vi "create test channels.vi"() -> (0 "error out":errorcluster, 1 "names":string[](array[string]), 2 "Array":refnum<class "EIP Tags Channel.lvclass">[](array[class]), 3 "EthernetIP configuration out":refnum<class "EIP Tags Configuration.lvclass">)   [LabVIEW 2013, in "EthernetIP tests.lvlib"]
uses:
  EthernetIP tests.lvlib
  channel/EIP Tags Channel.lvclass
  configuration/EIP Tags Configuration.lvclass
  configuration/eip tag types.ctl
  <vilib>/NI/Configuration Framework/serializable configuration/NISE_CEF_serializable configuration.lvclass
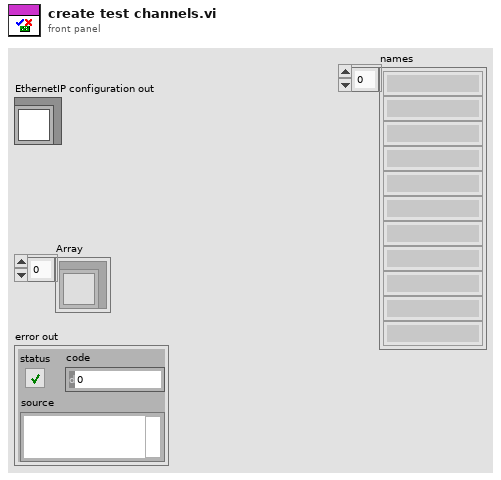
[diagram p1: front panel]
types:
  T1 = typedef "EIP Tags Configuration.lvclass/eip tag types.ctl" = enum16{"SINT", "INT", "DINT", "REAL", "BOOL", "STRING"}
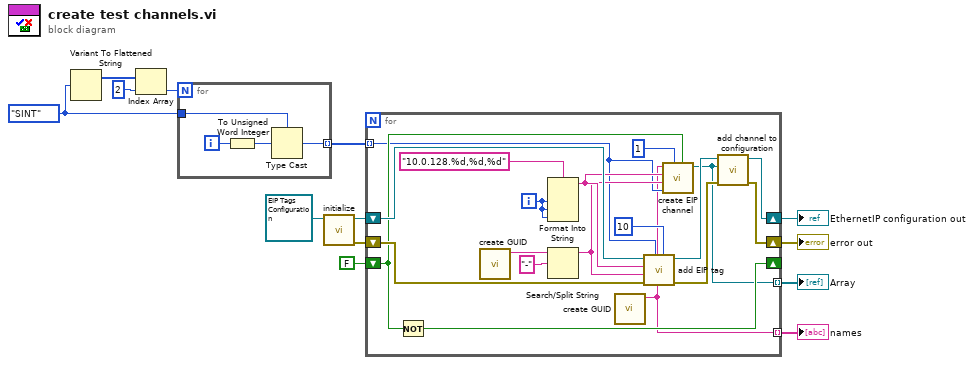
[diagram p0: block diagram]
diagram:
  w8 = eip_tag_types."SINT" ("eip tag types")
  n1 = Variant To Flattened String(Variant=w8) -> (1:w9:i16[])  [unwired: 1 out]
  n2 = Index Array(array=w9, index=2) -> (element=w11:i16)
  n3 = for {
    N: w11 -> [_]
    tunnel: [w16] -> w4 mode=indexing
    tunnel: w8 -> [w14]
    i -> [w17]
    n4 = To Unsigned Word Integer(number=w17) -> (unsigned 16bit integer=w15:u16)
    n5 = Type Cast(type=w14, x=w15) -> (*(type *) &x=w16:T1)
  }
  n6 = call <vilib>:"initialize.vi"("configuration in"=refnum<class "EIP Tags Configuration.lvclass"> refnum ("tag bus configurable plugin module configuration")) -> ("error out"=w5:errorcluster, "configuration out"=w6:refnum<class "EIP Tags Configuration.lvclass">)  [unwired: 8 in, 1 out]
  n7 = for {
    shift-right: [w26] -> w7
    shift-left: w6 -> [w34]
    shift-right: [w28] -> w13
    shift-left: w5 -> [w36]
    tunnel: w4 -> [w20] mode=indexing
    shift-right: [w25] -> _
    shift-left: FALSE ("output?") -> [w24]
    tunnel: [w19] -> w2 mode=indexing
    tunnel: [w18] -> w1 mode=indexing
    i -> [w32]
    n8 = Not(x=w24) -> (.not. x?=w25:bool)
    n9 = call <vilib>:"create GUID.vi"() -> ("uuid"=w30:string)  [unwired: 11 in]
    n10 = Format Into String(format string="10.0.128.%d,%d,%d", w32, w32, w32) -> (resulting string=w22:string)  [unwired: 2 in, 1 out]
    n11 = Search/Split String(string=w30, search string/char (-)="-") -> (substring before match=w21:string)  [unwired: 1 in, 2 out]
    n12 = call <vilib>:"create GUID.vi"() -> ("uuid"=w18:string)  [unwired: 11 in]
    n13 = call "add EIP tag.vi"("Number of Elements"=u32 10, "eip tag types"=w20, "error in"=w36, "Tag Name"=w21, "Network Path"=w22, "EIP Tags configuration in"=w34) -> ("error out"=w35:errorcluster, "EIP Tags configuration out"=w27:refnum<class "EIP Tags Configuration.lvclass">)  [unwired: 4 in]
    n14 = call "create EIP channel.vi"("output?"=w24, "element index"=1, "eip tag type"=w20, "Tag Name"=w21, "Network Path"=w22, "name"=w18) -> ("EthernetIP Channel out"=w19:refnum<class "EIP Tags Channel.lvclass">)  [unwired: 5 in]
    n15 = call "add channel to configuration.vi"("error in"=w35, "TBM channel in"=w19, "EthernetIP configuration in"=w27) -> ("error out"=w28:errorcluster, "EthernetIP configuration out"=w26:refnum<class "EIP Tags Configuration.lvclass">)  [unwired: 7 in]
  }
  "error out" <- w13
  "Array" <- w2
  "EthernetIP configuration out" <- w7
  "names" <- w1
